vi "ActionVIUI.vi"() -> ()   [LabVIEW 2019, in "ActionVI.lvclass"]
uses:
  ActionVI.lvclass
  <vilib>/NI/Configuration Framework/Node/NodeRef.ctl
  <vilib>/NI/Configuration Framework/Node/NISE_CEF_Node.lvclass
  <vilib>/NI/AMC/Message Queue.ctl
  <vilib>/NI/AMC/Message.ctl
  <vilib>/NI/Tools/Keyed Array/KeyedArray.ctl
  <vilib>/NI/Configuration Framework/Node/UserEventRef.ctl
  <vilib>/NI/Configuration Framework/Controls/EventCluster.ctl
  C:/Program Files (x86)/National Instruments/LabVIEW 2019/vi.lib/NI/Configuration Framework/Node/NISE_CEF_Node.lvclass
  ActionVI.lvclass/ActionVI.ctl
  Read Action VI Properties.vi
  Write Action VI Properties.vi
  <vilib>/NI/AMC/Create Single Message.vi
  <vilib>/NI/AMC/Update Message Routing Info.vi
  <vilib>/NI/AMC/Send Message.vi
  <vilib>/NI/AMC/AMC.lvlib
  Configuration Tool.lvlib
  <vilib>/NI/Tools/Keyed Array/Tools_KeyedArray.lvlib
  <vilib>/NI/Configuration Framework/NISE_CEF_TreeControl.lvlib
panel:
  in  "Main UI Tab":enum32{"Action VI"}(tab)
  in  "Host Path to ActionVI":path
  in  "user event":T1
  in  "main queue":T2
  in  "node ref":T3
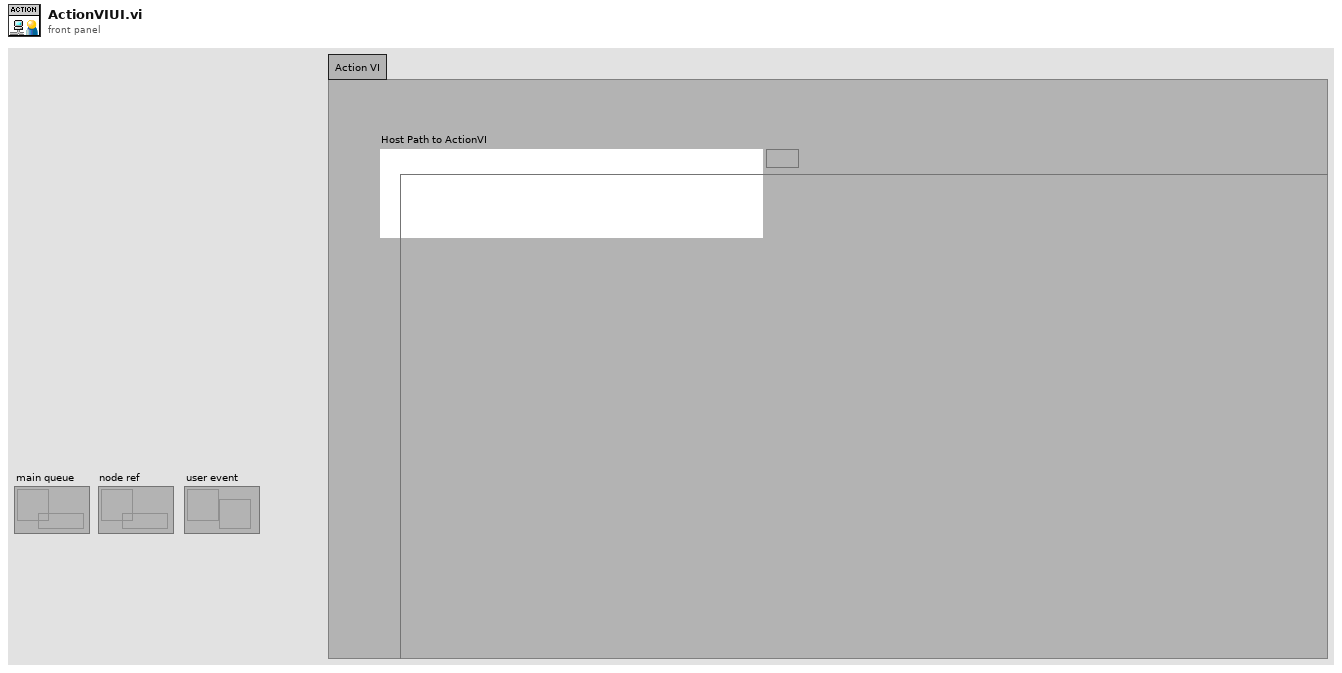
[diagram p1: front panel]
types:
  T1 = typedef "NISE_CEF_Node.lvclass/UserEventRef.ctl" = refnum<user-event>
  T2 = typedef "AMC.lvlib/Message Queue.ctl" = refnum<queue>
  T3 = typedef "NISE_CEF_Node.lvclass/NodeRef.ctl" = refnum<data-value>
  T4 = typedef "Path Cluster.ctl" = cluster{"Path":path, "Path Type":enum16{"Absolute", "To Base", "To Common Doc Dir", "To Application Data Dir"}}
  T5 = enum16{"Absolute", "To Base", "To Common Doc Dir", "To Application Data Dir"}
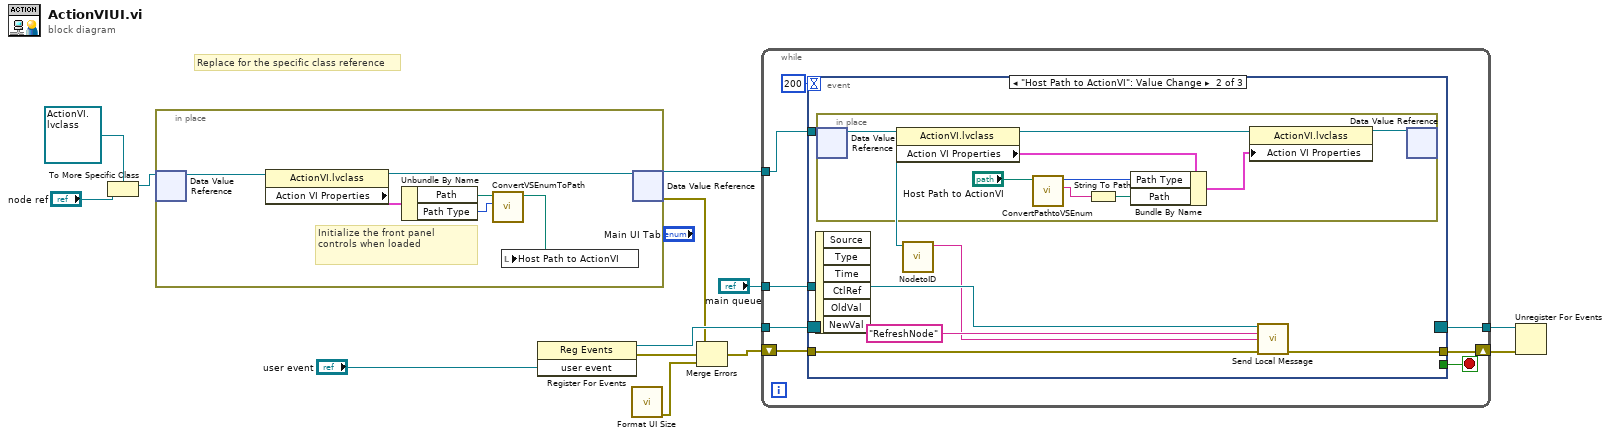
[diagram p0: block diagram]
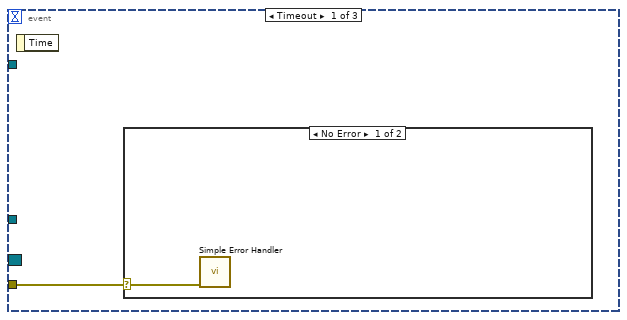
[diagram p2: hidden frame]
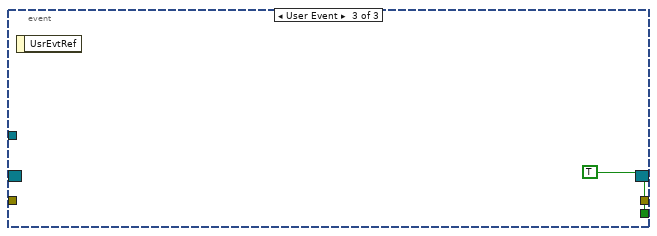
[diagram p4: hidden frame]
diagram:
  # "Replace for the specific class reference"
  n1 = To More Specific Class(target class=refnum<data-value> refnum ("data value reference"), reference="node ref") -> (specific class reference=w6:refnum<data-value>)  [unwired: 1 in, 1 out]
  n2 = in-place {
    # "Initialize the front panel controls when loaded"
    n3 = in-place-dvr #1(w6) -> (w19:refnum<class "ActionVI.lvclass">)  [unwired: 1 out]
    n4 = property class="ActionVI.lvclass"(reference=w19) -> (reference out=w18:refnum<class "ActionVI.lvclass">, "Action VI Properties"=w17:T4)  [unwired: 1 in, 1 out]
    n5 = Unbundle By Name(w17) -> ("Path"=w16:path, "Path Type"=w15:T5)
    n6 = call "ConvertVSEnumToPath.vi"("Source.Path Type"=w15, "Path In"=w16) -> ("appended path"=w14:path)  [unwired: 9 in]
    n7 = local write "Host Path to ActionVI"(w14) -> ()
    n8 = in-place-dvr #1(w18) -> (w13:refnum<data-value>, w3:errorcluster)
  }
  n9 = register-events("user event") -> (reference out=w10:refnum<event-registration>, error out=w4:errorcluster)  [unwired: 2 in]
  n10 = call "Format UI Size.vi"() -> ("error out"=w1:errorcluster)  [unwired: 11 in]
  n11 = Merge Errors(w3, w4, w1) -> (w2:errorcluster)
  n12 = while {
    tunnel: w13 -> [w27]
    tunnel: "main queue" -> [w26]
    tunnel: w10 -> [w24]
    tunnel: [w23] -> w9
    shift-right: [w21] -> w8
    shift-left: w2 -> [w20]
    stop <- w22 stop-if-true
    n13 = event shown="[1] \"Host Path to ActionVI\": Value Change" {
      selector: w24 -> [_ _ _]
      dyn-events: [_ _ _] -> w23
      timeout: 200 -> [_ _ _]
      tunnel: w27 -> [_ w33 _]
      tunnel: w26 -> [_ w34 _]
      tunnel: [_ _ TRUE] -> w22
      tunnel: [_ w31 _] -> w21
      tunnel: w20 -> [w28 w30 _]
      event Timeout {
        n14 = event-data() -> ()  [unwired: 1 in, 1 out]
        n15 = case shown="No Error" w28 {
          selector: w28 -> [w29 _]
          frame No Error {
            n16 = call <vilib>:"Simple Error Handler.vi"("error in (no error)"=w29) -> ()  [unwired: 4 in, 5 out]
          }
          frame Error {
          }
        }
      }
      event "Host Path to ActionVI": Value Change {
        n17 = event-data() -> ()  [unwired: 1 in, 6 out]
        n18 = in-place {
          n19 = in-place-dvr #2(w33) -> (w43:refnum<class "ActionVI.lvclass">)  [unwired: 1 out]
          n20 = property class="ActionVI.lvclass"(reference=w43) -> (reference out=w36:refnum<class "ActionVI.lvclass">, "Action VI Properties"=w42:T4)  [unwired: 1 in, 1 out]
          n21 = call "ConvertPathtoVSEnum.vi"("Path In"="Host Path to ActionVI") -> ("Remaining Path"=w40:string, "VS Enum Out"=w39:T5)  [unwired: 9 in]
          n22 = String To Path(string=w40) -> (path=w38:path)
          n23 = Bundle By Name(cluster=w42, "Path Type"=w39, "Path"=w38) -> (w41:T4)
          n24 = property class="ActionVI.lvclass"(reference=w36, "Action VI Properties"=w41) -> (reference out=w44:refnum<class "ActionVI.lvclass">)  [unwired: 1 in, 1 out]
          n25 = in-place-dvr #2(w44) -> ()  [unwired: 2 out]
        }
        n26 = call <vilib>:"NodetoID.vi"("node ref"=w33) -> ("ID"=w32:string)  [unwired: 9 in, 1 out]
        n27 = call <vilib>:"Send Local Message.vi"("message queue in"=w34, "message name"="RefreshNode" ("Message Name"), "message value"=w32, "error in"=w30) -> ("error out"=w31:errorcluster)  [unwired: 9 in, 2 out]
      }
      event User Event {
        n28 = event-data() -> ()  [unwired: 1 in, 1 out]
      }
    }
  }
  n29 = Unregister For Events(event registration refnum=w9, error in=w8) -> ()  [unwired: 1 out]
